vi "Check Cancel.vi"(11 "Repeat Message Control in":refnum<class "Repeat Message Control.lvclass">) -> (2 "Cancel":bool)   [LabVIEW 2020, in "Volatus.lvlib" / "Repeat Message Control.lvclass"]
uses:
  Repeat Message Control.lvclass
  Repeat Message Control.lvclass/Repeat Message Control.ctl
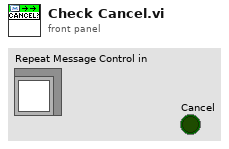
[diagram p1: front panel]
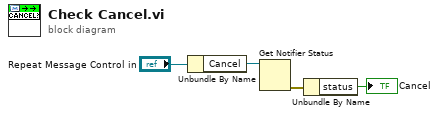
[diagram p0: block diagram]
diagram:
  n1 = Unbundle By Name("Repeat Message Control in") -> ("Cancel"=w3:refnum<notifier>)
  n2 = Get Notifier Status(notifier=w3) -> (error out=w2:errorcluster)  [unwired: 1 in, 4 out]
  n3 = Unbundle By Name(w2) -> ("status"=→"Cancel":bool)
